vi "BotPose Coords to Map Coords.vi"(11 "Point In":cluster{dbl, dbl}) -> (3 "Point Out":cluster{dbl, dbl})   [LabVIEW 2025]
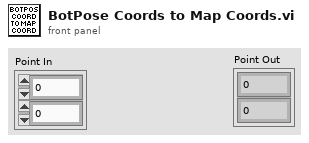
[diagram p1: front panel]
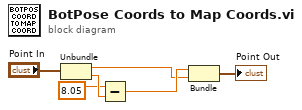
[diagram p0: block diagram]
diagram:
  n1 = Unbundle("Point In") -> (w1:dbl, w4:dbl)
  n2 = Subtract(x=8.05, y=w4) -> (x-y=w2:dbl)
  n3 = Bundle(w2, w1) -> (→"Point Out":cluster{dbl, dbl})  [unwired: 1 in]
